vi "Преобразование C в F_1.vi"(1 "Град C":dbl format="%.2f") -> (0 "Град F":dbl format="%.2f")   [LabVIEW 2017]
doc: "This VI is the solution to Exercise 3-1 from the LabVIEW Basics I Course. \n\nThis VI takes a number representing degrees Celsius and converts it to degrees Fahrenheit."
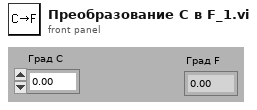
[diagram p1: front panel]
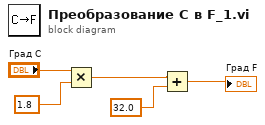
[diagram p0: block diagram]
diagram:
  n1 = Multiply(x="Град C", y=1.8) -> (x*y=w2:dbl)
  n2 = Add(x=w2, y=32.0) -> (x+y=→"Град F":dbl)
